vi "Bertta_v05.vi"() -> ()   [LabVIEW 2015]
uses:
  BERTTA.dll
panel:
  in  "Heidolph":dbl(slide) scale=0.0..1000.0
  in  "Ismatec":dbl(slide) scale=0.0..160.0
  in  "Tab Control":T1(tab)
  in  "Description":string
  in  "Project name":string
  in  "User (initials)":string
  out "Mettler":dbl(graph)
  out "?":dynamicdata(graph)
  in  "Balances":bool[](array[boolean])
  out "Waveform Chart 3":dynamicdata(graph)
  out "Table":string[][](table)
  in  "Headers":string[](array[string])
  in  "Seq":dbl[][](array[numeric])=[[20.0, 60.0, 40.0], [60.0, 40.0, 20.0], [100.0, 100.0, 100.0]]
  out "Elapsed":i32
  out "Step":i32
  in  "PAUSE":bool
  out "Sp":dbl
  out "T":dbl
  out "Tinit":dbl
  out "Tset":dbl
  out "tr":dbl
  out "Sp - Tset":i32
  out "Change":i32
  in  "START | STOP":bool
  out "Waveform Chart":dynamicdata(graph)
  out "Waveform Chart 2":dynamicdata(graph)
  out "Rate (g/s)":dbl
  out "Time (s)":dbl
  out "Target (g)":dbl
  in  "Seq 2":dbl[][](array[numeric])=[[20.0, 60.0, 40.0], [60.0, 40.0, 20.0], [100.0, 100.0, 100.0]]
  in  "PAM 1":bool
  out "Weight (S1)":dbl
  in  "enable amount":i32
  out "target reached":i32
  out "x/y":dbl
  out "bal_previous":i32
  out "Step 2":i32
  in  "?":T2(tab)
  in  "Device port":dbl=1.0
  out "Debug msg":dbl
  in  "Device port":dbl=20.0
  in  "Device port":i32=6
  in  "Device port":i32=15
  # "1"
  # "2"
  # "3"
  # "4"
  # "Step 1"
  # "Step 2"
  # "Step 3"
  # "Step 4"
  # "Tinit"
  # "Tset"
  # "tr"
  # "Step 1"
  # "Step 2"
  # "Step 3"
  # "Step 4"
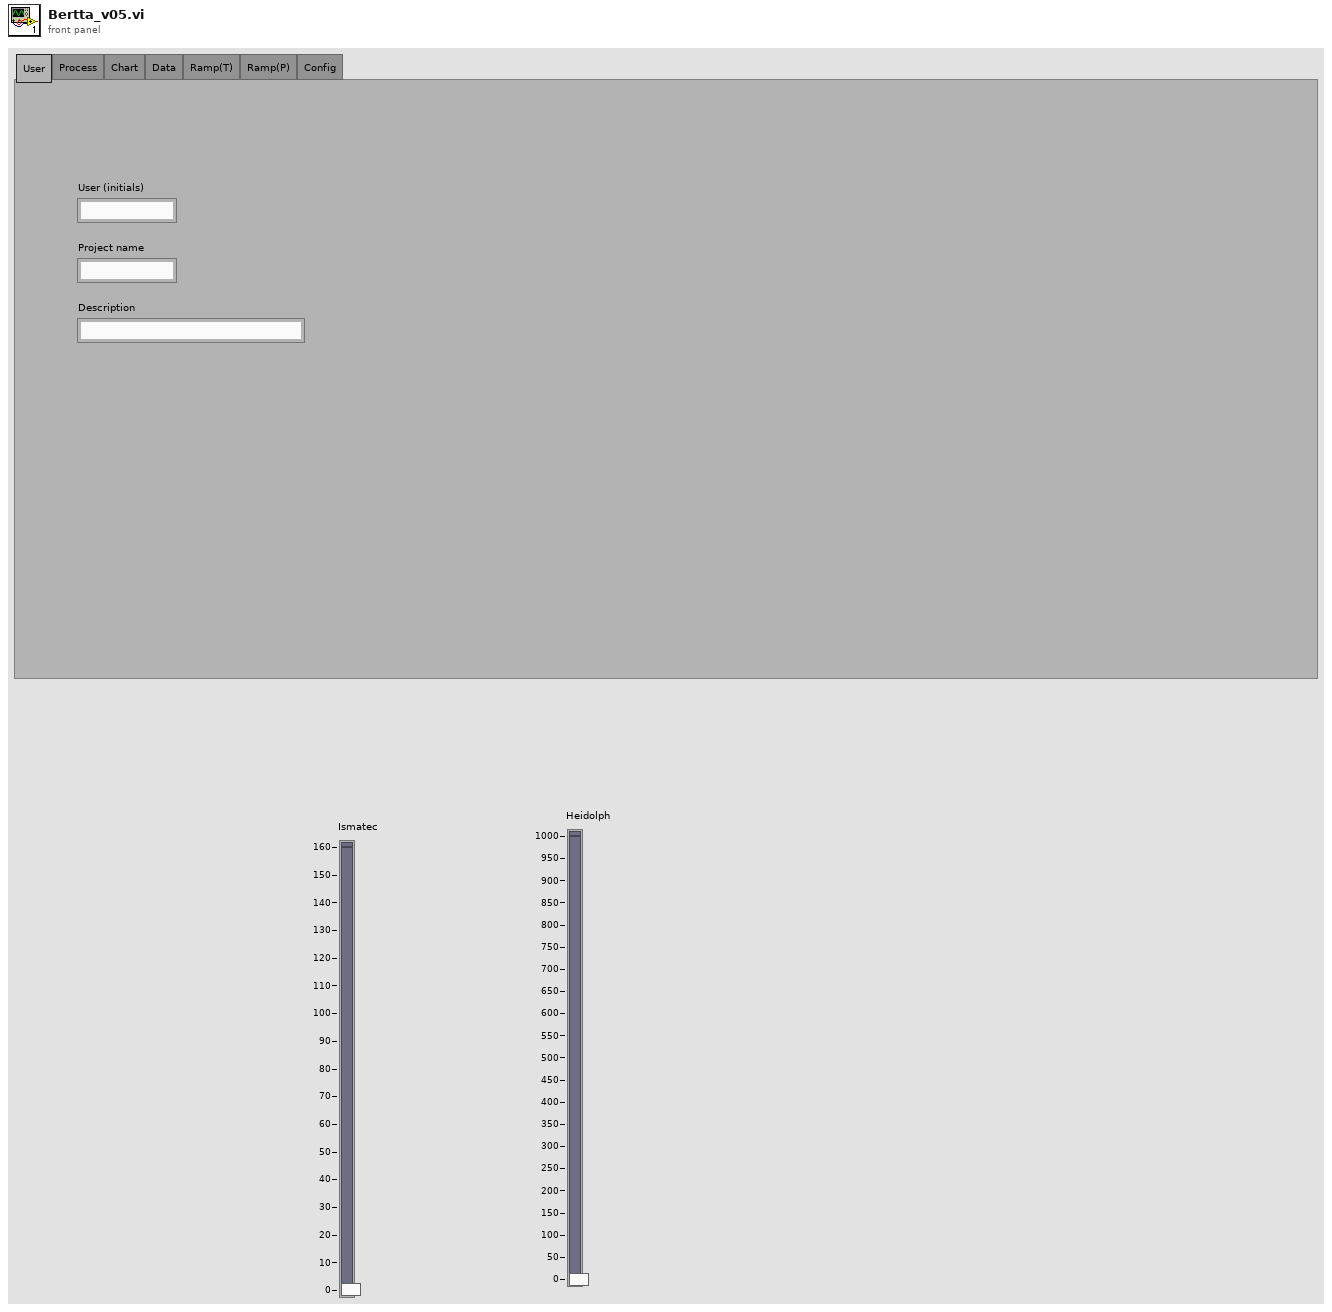
[diagram p1: front panel]
types:
  T1 = enum32{"User", "Process", "Chart", "Data", "Ramp(T)", "Ramp(P)", "Config"}
  T2 = enum32{"DB / File", "Lauda", "Heidolph", "Mettler 1", "Mettler 2", "Mettler 3", "Ismatec 1"}
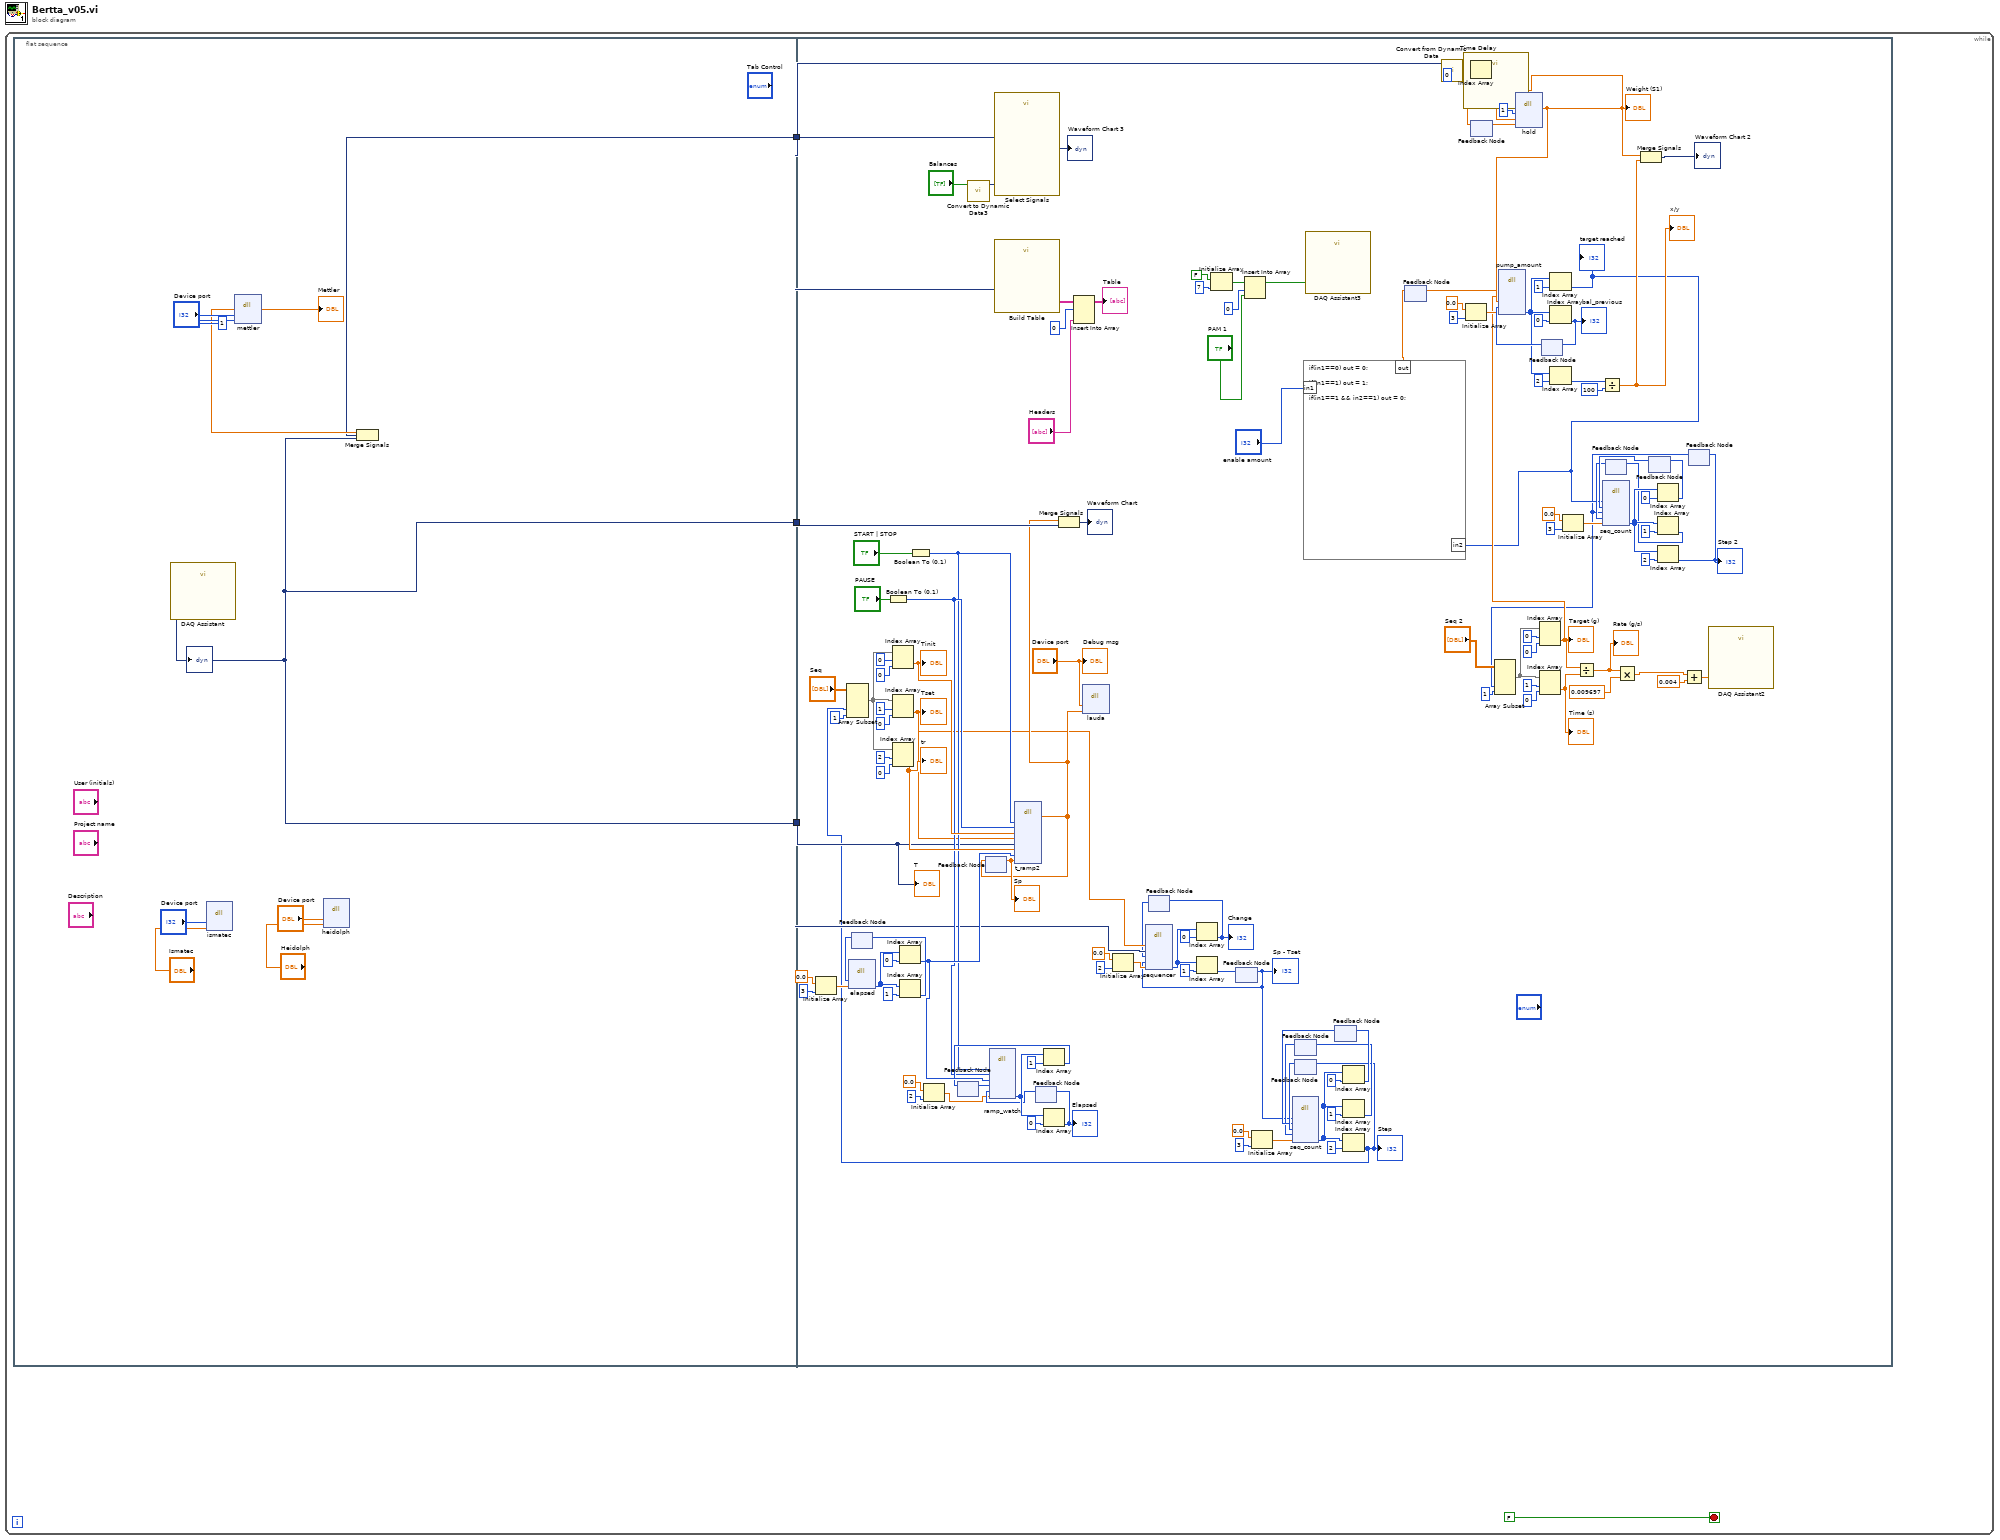
[diagram p0: block diagram]
diagram:
  n1 = while {
    stop <- FALSE stop-if-true
    n2 = flat-sequence {
      tunnel: [w5] -> w3
      tunnel: [w6] -> w2
      tunnel: [w6] -> w1
      tunnel: w3 -> [w50]
      tunnel: w2 -> [w95]
      tunnel: w1 -> [w122]
      frame #0 {
        n3 = call "DAQ Assistant"() -> ("data"=w6:dynamicdata)  [unwired: 17 in, 2 out]
        "?" <- w6
        n4 = dll-call lib="C:/Users/xlaraser/Documents/Visual Studio 2017/Projects/Bertta/BERTTA/Debug/BERTTA.dll" fn="ismatec"("port"="Device port", "speed"="Ismatec") -> ()  [unwired: 6 in, 2 out]
        n5 = dll-call lib="C:/Users/xlaraser/Documents/Visual Studio 2017/Projects/Bertta/BERTTA/Debug/BERTTA.dll" fn="mettler"("port"="Device port", "msg"=1) -> ("return type"=w7:dbl)  [unwired: 5 in, 2 out]
        "Mettler" <- w7
        n6 = dll-call lib="C:/Users/xlaraser/Documents/Visual Studio 2017/Projects/Bertta/BERTTA/Debug/BERTTA.dll" fn="heidolph"("port"="Device port", "speed"="Heidolph") -> ()  [unwired: 6 in, 2 out]
        n7 = Merge Signals(w7, w6) -> (w5:dynamicdata)
      }
      frame #1 {
        n8 = Initialize Array(0.0 ("element"), 3 ("dimension size")) -> (w133:dbl[])
        n9 = feedback #1() -> (w127:i32)  [unwired: 1 in]
        n10 = dll-call lib="C:/Users/xlaraser/Documents/Visual Studio 2017/Projects/Bertta/BERTTA/Debug/BERTTA.dll" fn="elapsed"("last_time"=w127, "params"=w133) -> ("params"=w109:i32[])  [unwired: 5 in, 2 out]
        n11 = Boolean To (0,1)(Boolean="PAUSE") -> (0, 1=w97:i16)
        n12 = Index Array(array=w109, index=0) -> (element=w108:i32)
        n13 = Index Array(array=w109, index=1) -> (element=w128:i32)
        n14 = feedback-in #1(w128) -> ()
        n15 = Boolean To (0,1)(Boolean="START | STOP") -> (0, 1=w96:i16)
        n16 = Initialize Array(0.0 ("element"), 2 ("dimension size")) -> (w98:dbl[])
        n17 = feedback #2() -> (w101:i32)  [unwired: 1 in]
        n18 = call "Convert to Dynamic Data3"("Array"="Balances") -> ("Dynamic Data Type"=w135:dynamicdata)  [unwired: 3 in]
        n19 = feedback #3() -> (w134:dbl)  [unwired: 1 in]
        "Sp" <- w134
        n20 = call "Select Signals"("Selector Input"=w135, "Signals"=w50) -> ("Signal Out"=→"Waveform Chart 3":dynamicdata)  [unwired: 8 in, 1 out]
        n21 = call "Build Table"("Signals"=w50) -> ("Table"=w138:string[][])  [unwired: 4 in, 6 out]
        n22 = feedback #4() -> (w103:i32)  [unwired: 1 in]
        n23 = dll-call lib="C:/Users/xlaraser/Documents/Visual Studio 2017/Projects/Bertta/BERTTA/Debug/BERTTA.dll" fn="ramp_watch"("enable"=w96, "pause"=w97, "elapsed"=w108, "elapsed_previous"=w101, "elapsed_total"=w103, "params"=w98) -> ("params"=w105:i32[])  [unwired: 9 in, 2 out]
        n24 = Index Array(array=w105, index=1) -> (element=w102:i32)
        n25 = feedback-in #2(w102) -> ()
        n26 = Index Array(array=w105, index=0) -> (element=w104:i32)
        "Elapsed" <- w104
        n27 = feedback-in #4(w104) -> ()
        n28 = Insert Into Array(array=w138, index (row)=0, new element="Headers") -> (→"Table":string[][])  [unwired: 1 in]
        n29 = Initialize Array(0.0 ("element"), 2 ("dimension size")) -> (w86:dbl[])
        n30 = feedback #5() -> (w89:i32)  [unwired: 1 in]
        n31 = Initialize Array(FALSE ("element"), 7 ("dimension size")) -> (w68:bool[])
        n32 = feedback #6() -> (w72:i32)  [unwired: 1 in]
        "Sp - Tset" <- w72
        n33 = Insert Into Array(array=w68, index=0, new element="PAM 1") -> (w65:bool[])
        n34 = Initialize Array(0.0 ("element"), 3 ("dimension size")) -> (w84:dbl[])
        n35 = feedback #7() -> (w75:i32)  [unwired: 1 in]
        n36 = feedback #8() -> (w77:i32)  [unwired: 1 in]
        n37 = call "DAQ Assistant3"("data"=w65) -> ()  [unwired: 17 in, 2 out]
        n38 = feedback #9() -> (w76:i32)  [unwired: 1 in]
        n39 = dll-call lib="C:/Users/xlaraser/Documents/Visual Studio 2017/Projects/Bertta/BERTTA/Debug/BERTTA.dll" fn="seq_count"("in1"=w72, "in2"=w76, "in3"=w77, "in4"=w75, "params"=w84) -> ("params"=w78:i32[])  [unwired: 8 in, 2 out]
        n40 = Index Array(array=w78, index=0) -> (element=w74:i32)
        n41 = feedback-in #9(w74) -> ()
        n42 = Index Array(array=w78, index=1) -> (element=w73:i32)
        n43 = feedback-in #7(w73) -> ()
        n44 = Index Array(array=w78, index=2) -> (element=w71:i32)
        "Step" <- w71
        n45 = Array Subset(array="Seq", index (col)=w71, length (col)=1 ("length")) -> (w115:dbl[][])  [unwired: 2 in]
        n46 = Index Array(array=w115, index (row)=0, index (col)=0 ("disabled index (col)")) -> (element=w114:dbl)
        "Tinit" <- w114
        n47 = Index Array(array=w115, index (row)=1, index (col)=0 ("disabled index (col)")) -> (element=w94:dbl)
        "Tset" <- w94
        n48 = Index Array(array=w115, index (row)=2, index (col)=0 ("disabled index (col)")) -> (element=w110:dbl)
        "tr" <- w110
        n49 = dll-call lib="C:/Users/xlaraser/Documents/Visual Studio 2017/Projects/Bertta/BERTTA/Debug/BERTTA.dll" fn="t_ramp2"("enable"=w96, "pause"=w97, "Tinit"=w114, "Tset"=w94, "Tcurrent"=w95, "ramp_time"=w110, "elapsed"=w108, "sp_old"=w134) -> ("return type"=w121:dbl)  [unwired: 11 in, 2 out]
        n50 = feedback-in #3(w121) -> ()
        n51 = Merge Signals(w121, w122) -> (→"Waveform Chart":dynamicdata)
        n52 = dll-call lib="C:/Users/xlaraser/Documents/Visual Studio 2017/Projects/Bertta/BERTTA/Debug/BERTTA.dll" fn="lauda"("port"="Device port", "set_temp"=w121) -> ()  [unwired: 6 in, 2 out]
        n53 = dll-call lib="C:/Users/xlaraser/Documents/Visual Studio 2017/Projects/Bertta/BERTTA/Debug/BERTTA.dll" fn="sequencer"("Tset"=w94, "Tcurrent"=w95, "treshold"=w89, "seq_previous"=w72, "params"=w86) -> ("params"=w91:i32[])  [unwired: 8 in, 2 out]
        n54 = Index Array(array=w91, index=0) -> (element=w90:i32)
        "Change" <- w90
        n55 = feedback-in #5(w90) -> ()
        n56 = Index Array(array=w91, index=1) -> (element=w85:i32)
        n57 = feedback-in #6(w85) -> ()
        n58 = feedback-in #8(w71) -> ()
        n59 = feedback #10() -> (w16:dbl)  [unwired: 1 in]
        n60 = call "Convert from Dynamic Data"("Dynamic Data Type"=w50) -> ("Array"=w51:dbl[])  [unwired: 3 in]
        n61 = Initialize Array(0.0 ("element"), 3 ("dimension size")) -> (w40:dbl[])
        n62 = Index Array(array=w51, index=0) -> (element=w49:dbl)
        n63 = feedback #11() -> (w48:dbl)  [unwired: 1 in]
        n64 = dll-call lib="C:/Users/xlaraser/Documents/Visual Studio 2017/Projects/Bertta/BERTTA/Debug/BERTTA.dll" fn="hold"("enable"=1, "in1"=w49, "in2"=w48) -> ("return type"=w37:dbl)  [unwired: 6 in, 2 out]
        "Weight (S1)" <- w37
        n65 = feedback-in #11(w37) -> ()
        n66 = feedback #12() -> (w43:i32)  [unwired: 1 in]
        n67 = Initialize Array(0.0 ("element"), 3 ("dimension size")) -> (w31:dbl[])
        n68 = feedback #13() -> (w23:i32)  [unwired: 1 in]
        n69 = feedback #14() -> (w24:i32)  [unwired: 1 in]
        n70 = feedback #15() -> (w14:i32)  [unwired: 1 in]
        n71 = Array Subset(array="Seq 2", index (col)=w14, length (col)=1 ("length")) -> (w62:dbl[][])  [unwired: 2 in]
        n72 = Index Array(array=w62, index (row)=0, index (col)=0 ("disabled index (col)")) -> (element=w35:dbl)
        "Target (g)" <- w35
        n73 = dll-call lib="C:/Users/xlaraser/Documents/Visual Studio 2017/Projects/Bertta/BERTTA/Debug/BERTTA.dll" fn="pump_amount"("enable"=w16, "target"=w35, "bal"=w37, "bal_previous"=w43, "params"=w40) -> ("params"=w38:i32[])  [unwired: 8 in, 2 out]
        n74 = Index Array(array=w62, index (row)=1, index (col)=0 ("disabled index (col)")) -> (element=w58:dbl)
        "Time (s)" <- w58
        n75 = Index Array(array=w38, index=1) -> (element=w19:i32)
        "target reached" <- w19
        n76 = formula code="if(in1==0) out = 0;\n\nif(in1==1) out = 1;\n\nif(in1==1 && in2==1) out = 0;"("in1"="enable amount", "in2"=w19) -> ("out"=w17:dbl)
        n77 = feedback-in #10(w17) -> ()
        n78 = Index Array(array=w38, index=0) -> (element=w44:i32)
        "bal_previous" <- w44
        n79 = feedback-in #12(w44) -> ()
        n80 = Index Array(array=w38, index=2) -> (element=w34:i32)
        n81 = Divide(x=w35, y=w58) -> (x/y=w57:dbl)
        "Rate (g/s)" <- w57
        n82 = Divide(x=w34, y=100) -> (x/y=w33:dbl)
        "x/y" <- w33
        n83 = dll-call lib="C:/Users/xlaraser/Documents/Visual Studio 2017/Projects/Bertta/BERTTA/Debug/BERTTA.dll" fn="seq_count"("in1"=w19, "in2"=w24, "in3"=w14, "in4"=w23, "params"=w31) -> ("params"=w25:i32[])  [unwired: 8 in, 2 out]
        n84 = Multiply(x=w57, y=0.009697) -> (x*y=w55:dbl)
        n85 = Merge Signals(w37, w33) -> (→"Waveform Chart 2":dynamicdata)
        n86 = Index Array(array=w25, index=0) -> (element=w22:i32)
        n87 = feedback-in #14(w22) -> ()
        n88 = Index Array(array=w25, index=1) -> (element=w21:i32)
        n89 = feedback-in #13(w21) -> ()
        n90 = Index Array(array=w25, index=2) -> (element=w15:i32)
        "Step 2" <- w15
        n91 = Add(x=w55, y=0.004) -> (x+y=w54:dbl)
        n92 = feedback-in #15(w15) -> ()
        n93 = call "DAQ Assistant2"("data"=w54) -> ()  [unwired: 17 in, 2 out]
        "T" <- w95
        "Debug msg" <- "Device port"
      }
    }
    n94 = call "Time Delay"() -> ()  [unwired: 11 in, 1 out]
  }
